vi "test_load_allmat_hyst_sat.vi"() -> ()   [LabVIEW 2017]
uses:
  <vilib>/Platform/TimedLoop/XDataNode/timing_clust.ctl
  <vilib>/Platform/TimedLoop/XDataNode/nitl_modes.ctl
  <vilib>/Platform/TimedLoop/XDataNode/wakeup.ctl
  <vilib>/rvi/Emulation/niFpgaGetClockAttributes.vi
  <vilib>/rvi/Emulation/niFpgaSctlEmulationGetInTimedLoop.vi
  <vilib>/rvi/Emulation/niFpgaEmulationReportErrorSimple.vi
  <vilib>/rvi/Emulation/niFpgaCriticalErrorInLSC.vi
  <vilib>/rvi/Memory/Memory_Emulation/nirvimemoryFastEmulation.vi
  <vilib>/rvi/Memory/Memory_Emulation/nirvimemoryEmulation.vi
  <vilib>/rvi/Emulation/niFpgaEmulationIsFPGAContextNoSignature.vi
  <vilib>/rvi/DataTransferAndStorage/Container/Common/niFpgaContainerGetUniqueNameForEmu.vi
  <vilib>/rvi/Emulation/niFpgaProcessEmulError.vi
  <vilib>/rvi/errors/nirviReportUnexpectedCaseInternalError (U32).vi
  <vilib>/Platform/TimedLoop/XDataNode/XDataNode.xnode
  <vilib>/rvi/DataTransferAndStorage/Container/XNode/niFpgaContainer.xnode
  <vilib>/Platform/TimedLoop/XDataNode/XDNodeRunTimeDep.lvlib
panel:
  out "L_fxp":fxp<+/-,16,5>[](array[numeric])
  out "K_fxp":fxp<+/-,16,5>[](array[numeric])
  in  "stop":bool
  out "sat_ds":fxp<+/-,16,5>[](array[numeric])
  out "sat_ws":fxp<+/-,16,5>[](array[numeric])
  out "hyst_rs":fxp<+/-,16,5>[](array[numeric])
  out "hyst_ws":fxp<+/-,16,5>[](array[numeric])
  in  "N_sat":u8
  in  "N_hyst":u8
  out "SS FIFO TimeOut?":bool
  in  "NS_O/C":u8=2
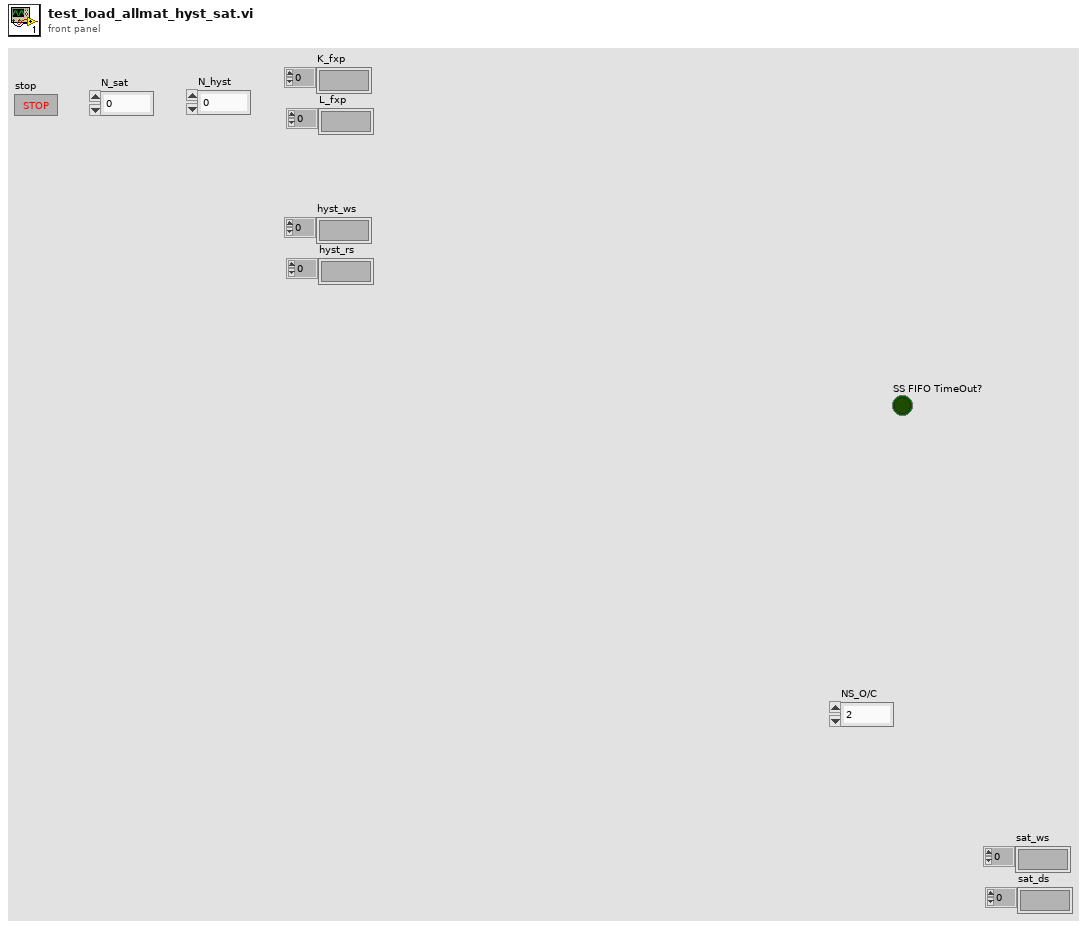
[diagram p1: front panel]
types:
  T1 = typedef "XDNodeRunTimeDep.lvlib/timing_clust.ctl" = cluster{"Expected End [f-1]":u64, "Actual End [f-1]":u64, "Finished Late? [f-1]":bool, "Expected End [i-1]":u64, "Actual End [i-1]":u64, "Finished Late? [i-1]":bool, "Expected Start [i]":u64, "Actual Start [i]":u64, "Expected Start [f]":u64, "Actual Start [f]":u64, "Source Name":string, "Structure Name":string, "Period":i64, "Deadline":i64, "Offset":i64, "Start":i64, "Priority":i32, "Timeout":i32, "Mode":T2, "Wakeup Reason":T3, "Error":errorcluster, "Source Type":string, "Secondary Source Type":string, "Global End Time":u64, "Global Start Time":u64, "Frame Duration":u64, "Iteration Duration":u64, "Assigned CPU":i32, "I/O Scan Engine Mode":u32}
  T2 = typedef "XDNodeRunTimeDep.lvlib/nitl_modes.ctl" = enum32{"No Change", "Process missed periods, maintain original phase", "Discard missed periods, maintain original phase", "Process missed periods, ignore original phase", "Discard missed periods, ignore original phase"}
  T3 = typedef "XDNodeRunTimeDep.lvlib/wakeup.ctl" = enum32{"Normal", "Aborted", "Asynchronous wakeup", "Timing source error", "Timed loop error", "Timeout"}
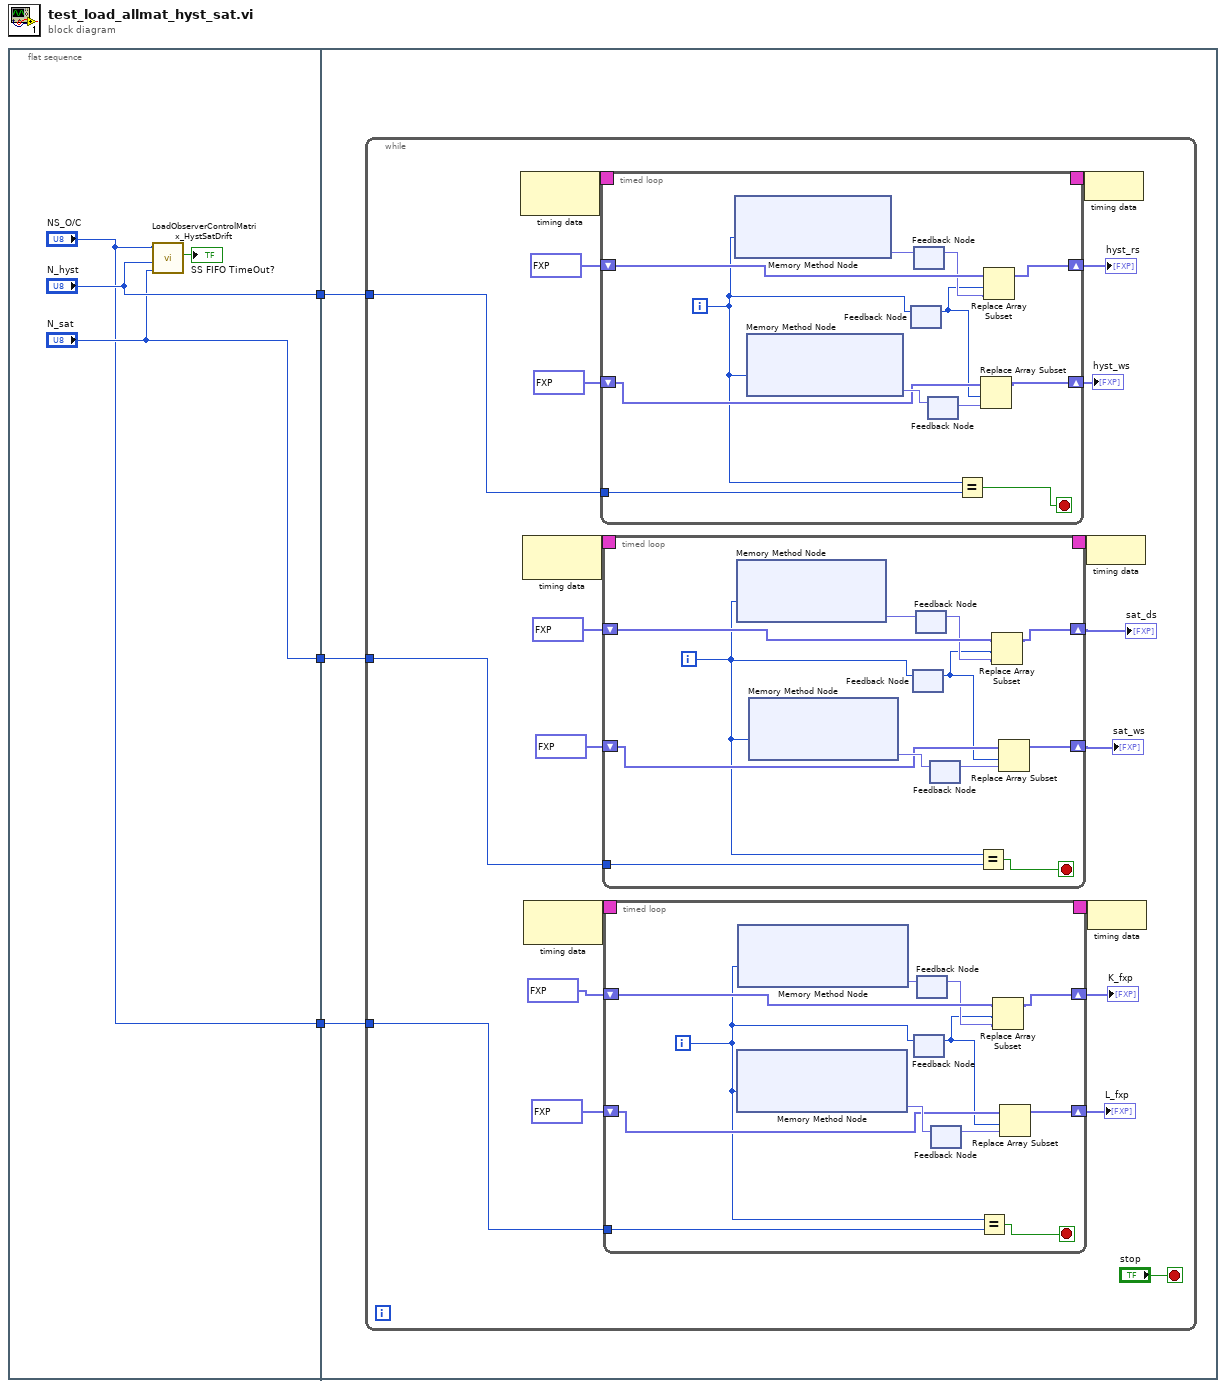
[diagram p0: block diagram]
diagram:
  n1 = flat-sequence {
    tunnel: ["N_hyst"] -> w3
    tunnel: ["N_sat"] -> w2
    tunnel: ["NS_O/C"] -> w1
    tunnel: w3 -> [w9]
    tunnel: w2 -> [w10]
    tunnel: w1 -> [w8]
    frame #0 {
      n2 = call "LoadObserverControlMatrix_HystSatDrift.vi"("Nsat"="N_sat", "Nhyst"="N_hyst", "NS_obs/cntrl"="NS_O/C") -> ("SS FIFO TimeOut?"=→"SS FIFO TimeOut?":bool)  [unwired: 8 in]
    }
    frame #1 {
      n3 = while {
        tunnel: w10 -> [w28]
        tunnel: w9 -> [w23]
        tunnel: w8 -> [w15]
        stop <- "stop" stop-if-true
        n4 = node-c288() -> (w30:T1)  [unwired: 1 in]
        n5 = node-c288() -> (w32:T1)  [unwired: 1 in]
        n6 = node-c288() -> (w17:T1)  [unwired: 1 in]
        n7 = timed-loop {
          timing: w30 -> [_]
          timing-out: [_] -> w29
          tunnel: w23 -> [w49]
          shift-right: [w56] -> w21
          shift-left: fxp<+/-,16,5>[] [0.0, 0.0, 0.0, 0.0, 0.0, 0.0, 0.0, 0.0, 0.0, 0.0, 0.0, 0.0] -> [w57]
          shift-right: [w54] -> w22
          shift-left: fxp<+/-,16,5>[] [0.0, 0.0, 0.0, 0.0, 0.0, 0.0, 0.0, 0.0, 0.0, 0.0, 0.0, 0.0] -> [w53]
          i -> [w50]
          stop <- w58 stop-if-true
          n8 = xnode ("Memory Method Node")("Address"=w50) -> ("Data"=w60:fxp<+/-,16,5>)  [unwired: 1 in, 1 out]
          n9 = xnode ("Memory Method Node")("Address"=w50) -> ("Data"=w59:fxp<+/-,16,5>)  [unwired: 1 in, 1 out]
          n10 = feedback #1() -> (w52:i32)  [unwired: 1 in]
          n11 = feedback-in #1(w50) -> ()
          n12 = feedback #2() -> (w55:fxp<+/-,16,5>)  [unwired: 1 in]
          n13 = feedback-in #2(w60) -> ()
          n14 = feedback #3() -> (w51:fxp<+/-,16,5>)  [unwired: 1 in]
          n15 = feedback-in #3(w59) -> ()
          n16 = Equal?(x=w50, y=w49) -> (x = y?=w58:bool)
          n17 = Replace Array Subset(array=w53, new element=w51, index=w52) -> (w54:fxp<+/-,16,5>[])
          n18 = Replace Array Subset(array=w57, new element=w55, index=w52) -> (w56:fxp<+/-,16,5>[])
        }
        "hyst_ws" <- w22
        "hyst_rs" <- w21
        n19 = timed-loop {
          timing: w32 -> [_]
          timing-out: [_] -> w31
          tunnel: w28 -> [w65]
          shift-right: [w71] -> w20
          shift-left: fxp<+/-,16,5>[] [0.0, 0.0, 0.0, 0.0, 0.0, 0.0, 0.0, 0.0, 0.0, 0.0, 0.0, 0.0] -> [w73]
          shift-right: [w70] -> w19
          shift-left: fxp<+/-,16,5>[] [0.0, 0.0, 0.0, 0.0, 0.0, 0.0, 0.0, 0.0, 0.0, 0.0, 0.0, 0.0] -> [w69]
          i -> [w66]
          stop <- w74 stop-if-true
          n20 = xnode ("Memory Method Node")("Address"=w66) -> ("Data"=w76:fxp<+/-,16,5>)  [unwired: 1 in, 1 out]
          n21 = xnode ("Memory Method Node")("Address"=w66) -> ("Data"=w75:fxp<+/-,16,5>)  [unwired: 1 in, 1 out]
          n22 = feedback #4() -> (w68:i32)  [unwired: 1 in]
          n23 = feedback-in #4(w66) -> ()
          n24 = feedback #5() -> (w72:fxp<+/-,16,5>)  [unwired: 1 in]
          n25 = feedback-in #5(w76) -> ()
          n26 = feedback #6() -> (w67:fxp<+/-,16,5>)  [unwired: 1 in]
          n27 = feedback-in #6(w75) -> ()
          n28 = Equal?(x=w66, y=w65) -> (x = y?=w74:bool)
          n29 = Replace Array Subset(array=w73, new element=w72, index=w68) -> (w71:fxp<+/-,16,5>[])
          n30 = Replace Array Subset(array=w69, new element=w67, index=w68) -> (w70:fxp<+/-,16,5>[])
        }
        "sat_ws" <- w19
        "sat_ds" <- w20
        n31 = timed-loop {
          timing: w17 -> [_]
          timing-out: [_] -> w16
          tunnel: w15 -> [w33]
          shift-right: [w39] -> w12
          shift-left: fxp<+/-,16,5>[] [0.0, 0.0, 0.0, 0.0, 0.0, 0.0, 0.0, 0.0, 0.0, 0.0, 0.0, 0.0, 0.0, 0.0, 0.0, 0.0, 0.0, 0.0, 0.0, 0.0, 0.0, 0.0, 0.0, 0.0] -> [w41]
          shift-right: [w38] -> w11
          shift-left: fxp<+/-,16,5>[] [0.0, 0.0, 0.0, 0.0, 0.0, 0.0, 0.0, 0.0, 0.0, 0.0, 0.0, 0.0, 0.0, 0.0, 0.0, 0.0, 0.0, 0.0, 0.0, 0.0, 0.0, 0.0, 0.0, 0.0] -> [w37]
          i -> [w34]
          stop <- w42 stop-if-true
          n32 = xnode ("Memory Method Node")("Address"=w34) -> ("Data"=w43:fxp<+/-,32,3>)  [unwired: 1 in, 1 out]
          n33 = xnode ("Memory Method Node")("Address"=w34) -> ("Data"=w44:fxp<+/-,32,10>)  [unwired: 1 in, 1 out]
          n34 = feedback #7() -> (w36:i32)  [unwired: 1 in]
          n35 = feedback-in #7(w34) -> ()
          n36 = feedback #8() -> (w40:fxp<+/-,32,10>)  [unwired: 1 in]
          n37 = feedback-in #8(w44) -> ()
          n38 = feedback #9() -> (w35:fxp<+/-,32,3>)  [unwired: 1 in]
          n39 = feedback-in #9(w43) -> ()
          n40 = Equal?(x=w34, y=w33) -> (x = y?=w42:bool)
          n41 = Replace Array Subset(array=w41, new element=w40, index=w36) -> (w39:fxp<+/-,16,5>[])
          n42 = Replace Array Subset(array=w37, new element=w35, index=w36) -> (w38:fxp<+/-,16,5>[])
        }
        "K_fxp" <- w12
        "L_fxp" <- w11
        n43 = node-c288(w29) -> ()
        n44 = node-c288(w31) -> ()
        n45 = node-c288(w16) -> ()
      }
    }
  }
